vi "QueryGrating.vi"(8 "error in (no error)":errorcluster, 11 "DongWoo in":refnum<class "DongWoo.lvclass">) -> (0 "error out":errorcluster, 3 "DongWoo out":refnum<class "DongWoo.lvclass">)   [LabVIEW 2023, in "DongWoo_Spectrometer.lvlib" / "DongWoo.lvclass"]
uses:
  DongWoo.lvclass
  DongWoo.lvclass/DongWoo.ctl
  Interfaces/AbstractInstrumentClasses/Spectrometers_LV/SpectrometerComm Messages/GratingChanged Msg/GratingChanged Msg.lvclass
  <vilib>/ActorFramework/Actor/Actor.lvclass
  C:/Program Files/National Instruments/LabVIEW 2023/vi.lib/ActorFramework/Actor/Actor.lvclass
  C:/Users/DELL/Documents/LVDAQ/ConcreteClasses/ConcreteInstrumentClasses/SpectrometerClasses/DongWoo_LV/DongWoo/DongWoo.lvclass
  C:/Users/DELL/Documents/LVDAQ/Interfaces/InitDeinitInterface/InitDeinit/InitDeinit.lvclass
  C:/Users/DELL/Documents/LVDAQ/Interfaces/AbstractInstrumentClasses/Spectrometers_LV/SpectrometerInterface/Spectrometer.lvclass
panel:
  in  "Bytes to Read":u32=54
  out "Numeric":i32
  in  "CW":string="CW"
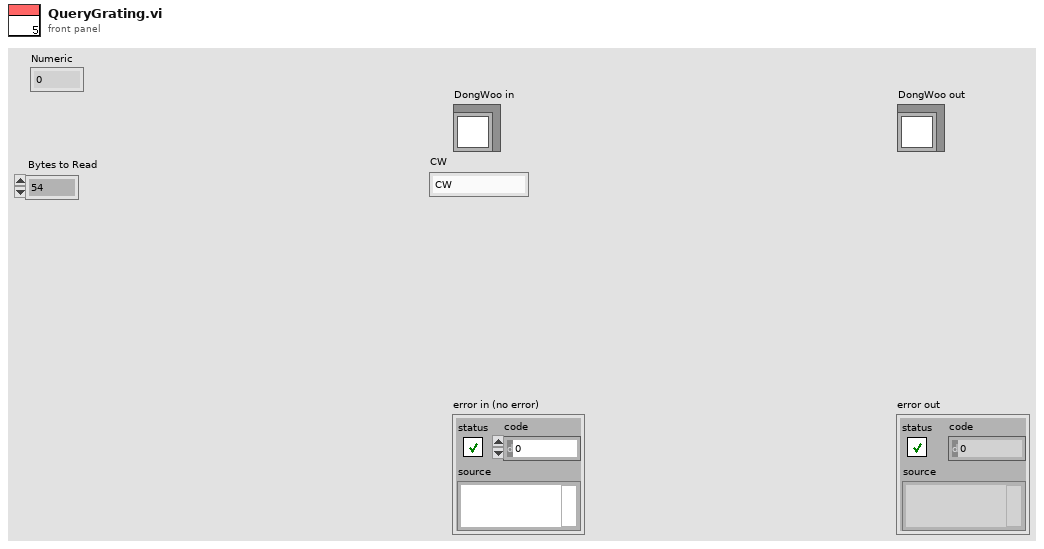
[diagram p1: front panel]
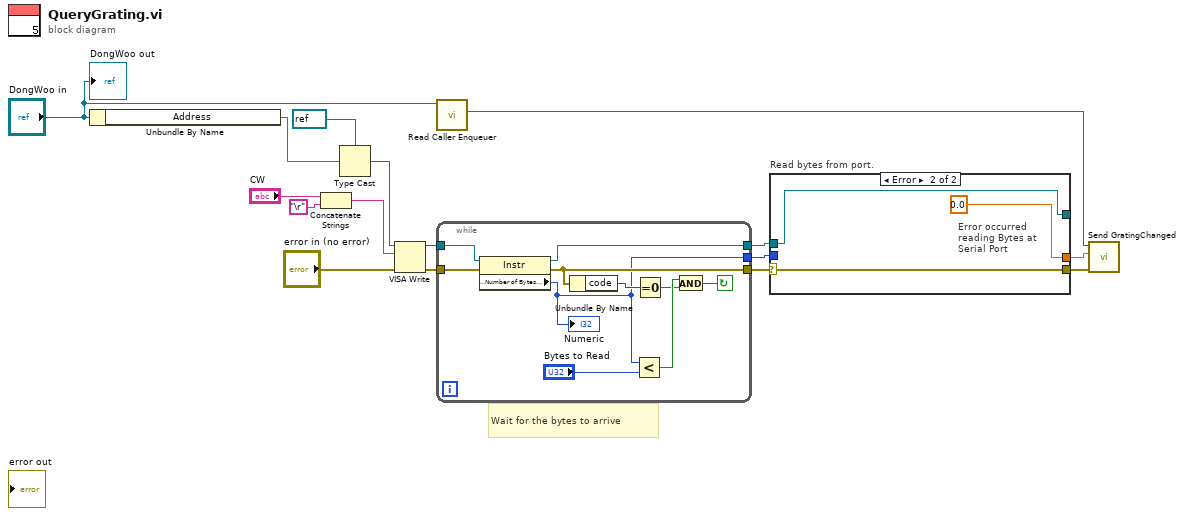
[diagram p0: block diagram]
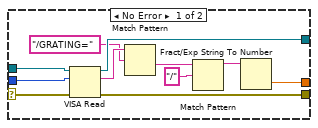
[diagram p2: hidden frame]
diagram:
  # "Wait for the bytes to arrive"
  n1 = Unbundle By Name("DongWoo in") -> ("Address"=w8:string)
  n2 = Concatenate Strings("CW", "\r") -> (w16:string)
  n3 = Type Cast(type=refnum<visa-resource-name> refnum ("VISA resource name"), x=w8) -> (*(type *) &x=w6:refnum<visa-resource-name>)
  n4 = VISA Write(VISA resource name=w6, write buffer=w16, error in (no error)="error in (no error)") -> (VISA resource name out=w10:refnum<visa-resource-name>, error out=w9:errorcluster)  [unwired: 1 out]
  n5 = call <vilib>:"Read Caller Enqueuer.vi"("Actor"="DongWoo in") -> ("Caller Enqueuer"=w4:refnum<class "Message Enqueuer.lvclass">)  [unwired: 10 in]
  n6 = while {
    tunnel: [w19] -> w11
    tunnel: [w17] -> w12
    tunnel: w10 -> [w25]
    tunnel: w9 -> [w20]
    tunnel: [w26] -> w13
    stop <- w22 continue-if-true
    n7 = property class="Instr"(reference=w25, error in=w20) -> (reference out=w26:refnum<visa-resource-name>, error out=w19:errorcluster, "Serial Settings:Number of Bytes at Serial Port"=w17:u32)
    "Numeric" <- w17
    n8 = Unbundle By Name(w19) -> ("code"=w21:i32)
    n9 = Less?(x=w17, y="Bytes to Read") -> (x < y?=w24:bool)
    n10 = Equal To 0?(x=w21) -> (x = 0?=w23:bool)
    n11 = And(x=w24, y=w23) -> (x .and. y?=w22:bool)
  }
  n12 = case "Read bytes from port." shown="Error" w11 {
    selector: w11 -> [w34 w39]
    tunnel: [w37 w39] -> w2
    tunnel: w13 -> [w36 w40]
    tunnel: w12 -> [w35 _]
    tunnel: [w33 w40] -> _
    tunnel: [w27 0.0] -> w1
    frame No Error {
      n13 = VISA Read(VISA resource name=w36, byte count=w35, error in (no error)=w34) -> (VISA resource name out=w33:refnum<visa-resource-name>, read buffer=w30:string, error out=w37:errorcluster)  [unwired: 1 out]
      n14 = Match Pattern(string=w30, regular expression="/GRATING=") -> (after substring=w31:string)  [unwired: 1 in, 3 out]
      n15 = Match Pattern(string=w31, regular expression="/") -> (before substring=w28:string)  [unwired: 1 in, 3 out]
      n16 = Fract/Exp String To Number(string=w28) -> (number=w27:dbl)  [unwired: 3 in, 1 out]
    }
    frame Error {
      # "Error occurred \nreading Bytes at \nSerial Port"
    }
  }
  n17 = call "Send GratingChanged.vi"("error in (no error)"=w2, "Grating"=w1, "Message Enqueuer"=w4) -> ()  [unwired: 7 in, 2 out]
  "DongWoo out" <- "DongWoo in"
